vi "Change Octave Working Path.vi"(7 "Measurement path in":path=path "D:/martin/WAC/WACsw - github/control_software/Filter function meter/Template/Example of FF meter template_data/FF_calibration_template_line_0010/session.info", 8 "error in (no error)":errorcluster) -> (0 "error out":errorcluster)   [LabVIEW 2020]
doc: "Change octave path, add paths to WAC data processing."
uses:
  Globals for GOLPI.vi
  external libraries/GOLPI 0.7.3.1 source distribution LV 20.0 32 bit/GOLPI library.lvlib
panel:
  out "command\n(for debug)":string="addpath('info'); addpath('qwtb'); qwtb_exec_algorithm('%s', 0, 1); disp('FINISHEDCR')"
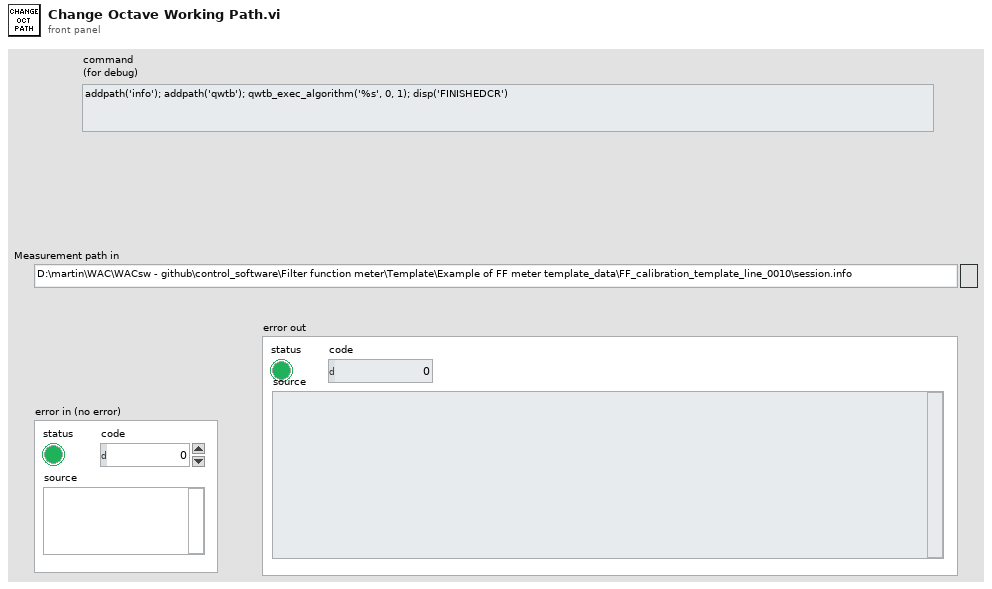
[diagram p1: front panel]
types:
  T1 = typedef "GOLPI library.lvlib/GOLPI reference Type Def.ctl" = cluster{"pipe handle":T2, "fast read timeout [ms]":u32, "fast read settle time [ms]":u32, "fast read to multiple [ms]":u32, "max elements per input line":u32, "slow read timeout [ms]":u32, "stdin double format specifier":string, "max elements per stdout output column":u32, "console mode bitstream":bool, "bitstream first read timeout [ms]":u32, "bitstream read timeout [ms]":u32, "struct transfer possible":bool, "matlab mode":bool}
  T2 = typedef "LV Process library.lvlib/Pipe Handle.ctl" = cluster{"lv_proc.dll file path":path, "process instance handle":u32[], "debug mode":bool, "debug data":cluster{"time":timestamp, "stdin":bool, "data":string}[]}
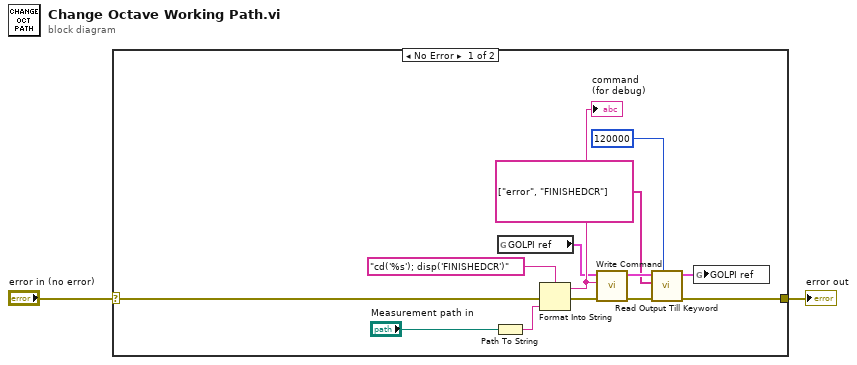
[diagram p0: block diagram]
diagram:
  n1 = case shown="No Error" "error in (no error)" {
    selector: "error in (no error)" -> [w5 w16]
    tunnel: [w6 w16] -> w2
    frame No Error {
      n2 = Path To String(path="Measurement path in") -> (string=w13:string)
      n3 = global read "Globals for GOLPI.vi" "GOLPI ref"() -> (w4:T1)
      n4 = Format Into String(format string="cd('%s'); disp('FINISHEDCR')", error in=w5, w13) -> (resulting string=w7:string, error out=w12:errorcluster)  [unwired: 1 in]
      "command\n(for debug)" <- w7
      n5 = call "Write Command.vi"("error in"=w12, "command"=w7, "GOLPI ref. in"=w4) -> ("error out"=w11:errorcluster, "GOLPI ref. out"=w10:T1)  [unwired: 7 in]
      n6 = call "Read Output Till Keyword.vi"("timeout [ms]"=u32 120000, "error in"=w11, "keywords"=string[] ["error", "FINISHEDCR"], "GOLPI ref. in"=w10) -> ("error out"=w6:errorcluster, "GOLPI ref. out"=w3:T1)  [unwired: 4 in, 2 out]
      n7 = global write "Globals for GOLPI.vi" "GOLPI ref"(w3) -> ()
    }
    frame Error {
    }
  }
  "error out" <- w2
